vi "ErrorMessageFromErrorCluster.vi"(10 "Error":errorcluster) -> (2 "Error Message":string)   [LabVIEW 2017, in "Assertion.Tests.lvlib"]
uses:
  Assertion.Tests.lvlib
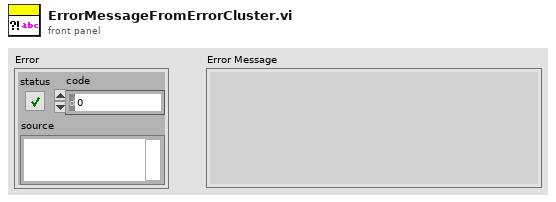
[diagram p1: front panel]
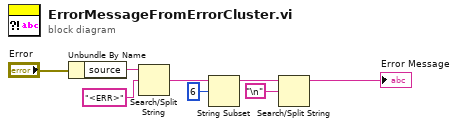
[diagram p0: block diagram]
diagram:
  n1 = Unbundle By Name("Error") -> ("source"=w6:string)
  n2 = Search/Split String(string=w6, search string/char (-)="<ERR>") -> (match + rest of string=w3:string)  [unwired: 1 in, 2 out]
  n3 = String Subset(string=w3, offset (0)=6) -> (substring=w2:string)  [unwired: 1 in]
  n4 = Search/Split String(string=w2, search string/char (-)="\n") -> (substring before match=→"Error Message":string)  [unwired: 1 in, 2 out]
